vi "dvp Vi Get Inverse State.vi"(10 "pInverseState":i32, 11 "handle":u32) -> (2 "pInverseState out":i32, 3 "function return":u32(ring))   [LabVIEW 2018, in "LabViewDVPCamera.lvlib"]
doc: "LabviewDvp2Api dvpStatus dvpViGetInverseState(dvpHandle handle, BOOL *pInverseState);"
uses:
  LabViewDVPCamera.lvlib
  LabViewDVPCamera/LabViewDVPCamera.dll
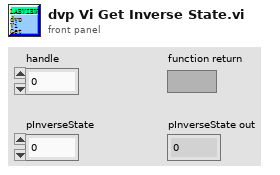
[diagram p1: front panel]
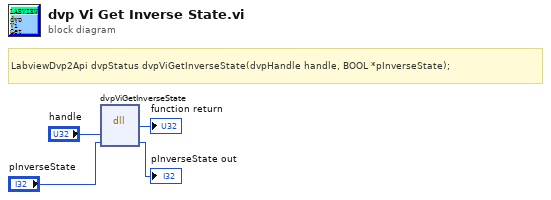
[diagram p0: block diagram]
diagram:
  # "LabviewDvp2Api dvpStatus dvpViGetInverseState(dvpHandle handle, BOOL *pInverseState);"
  n1 = dll-call lib="C:/Program Files (x86)/DVP2 Labview cn 64/Sample/LabViewDVPCamera/LabViewDVPCamera.*" fn="dvpViGetInverseState"("handle"="handle", "pInverseState"="pInverseState") -> (→"function return":u32, "pInverseState"=→"pInverseState out":i32)  [unwired: 4 in, 2 out]
